vi "3D Surface Graph.vi"() -> ()   [LabVIEW 2014]
doc: "本VI说明了三维曲面的使用方式。"
uses:
  <vilib>/Math Plots/3D Math Plots/3D Surface/3D Surface XCtrl/3D Surface.xctl
  <vilib>/Math Plots/3D Math Plots/3D Mesh/3D Mesh XCtrl/3D Mesh.xctl
  <vilib>/Math Plots/3D Math Plots/3D Contour/3D Contour XCtrl/3D Contour.xctl
  <vilib>/Math Plots/3D Math Plots/3D Contour/3D Contour Datatype/Public/Plot Helper (Vector).vi
  <vilib>/Math Plots/3D Math Plots/3D Mesh/3D Mesh Datatype/Public/Plot Helper (Vector).vi
  <vilib>/Math Plots/3D Math Plots/3D Surface/3D Surface Datatype/Public/Plot Helper (Vector).vi
  <vilib>/imath/engines/lvmath2/RunTimeEngine/Managers/WorkSpace/UID Generator.vi
  <vilib>/imath/engines/lvmath2/RunTimeEngine/BuiltInFunctions/max/1 input/NIMS_max(RV).vi
  <instcachedir>/0/NIMS_max(RV)_237633DB1D604D5BA7001287DF3C7957.lvgen/NIMS_max(RV)_237633DB1D604D5BA7001287DF3C7957_002.vi
  <vilib>/imath/engines/lvmath2/RunTimeEngine/BuiltInFunctions/min/1 input/NIMS_min(RV).vi
  <instcachedir>/0/NIMS_min(RV)_EE2DD3E2888846108C5160A664B67832.lvgen/NIMS_min(RV)_EE2DD3E2888846108C5160A664B67832_002.vi
  <vilib>/imath/engines/lvmath2/RunTimeEngine/BuiltInFunctions/linramp/NIMS_linramp.vi
  <vilib>/imath/engines/lvmath2/RunTimeEngine/BuiltInFunctions/meshgrid2d/NIMS_meshgrid2d(V,V).vi
  <instcachedir>/0/NIMS_meshgrid2d(V,V)_3733343E1C554A708015CFB0432C6A59.lvgen/NIMS_meshgrid2d(V,V)_3733343E1C554A708015CFB0432C6A59_000.vi
  <vilib>/imath/engines/lvmath2/RunTimeEngine/BuiltInFunctions/intrp2d_uneven/NIMS_[1o]_intrp2d_uneven.vi
  <vilib>/imath/engines/lvmath2/RunTimeEngine/RunTimeType/NIMS_RunTimeType_From StrictType (excl LVString).vi
  <instcachedir>/0/NIMS_RunTimeType_From StrictType (excl LVString)_15A5391EEA9C4AACB9955AC755B83D29.lvgen/NIMS_RunTimeType_From StrictType (excl LVString)_15A5391EEA9C4AACB9955AC755B83D29_000.vi
  <vilib>/imath/engines/lvmath2/RunTimeEngine/ErrorHandling/NIMS_Error From Error Code.vi
  <vilib>/imath/engines/lvmath2/RunTimeEngine/LocalVariableDefStatement/MC_LocalVariableDefStatement_Display.vi
  <vilib>/imath/engines/lvmath2/RunTimeEngine/BuiltInFunctions/mesh/NIMS_mesh(RM, RM).vi
  <vilib>/imathl/engines/lvmath/Functions/Error Handling/Create Error.vi
  <vilib>/imath/engines/lvmath2/RunTimeEngine/BuiltInFunctions/grid/NIMS_grid(Enums).vi
  <vilib>/imath/engines/lvmath2/RunTimeEngine/Managers/SymbolTable/Clear UID.vi
  <vilib>/imath/engines/lvmath2/RunTimeEngine/ErrorHandling/NIMS_Finalize Error.vi
  <vilib>/Math Plots/3D Math Plots/3D Surface/3D Surface Datatype/3D Surface Datatype.lvclass
  <vilib>/imath/engines/lvmath2/RunTimeEngine/RangeToken/NIMS_Range_R2 - Integer.vi
  <vilib>/imath/engines/lvmath2/RunTimeEngine/IndexRead/NIMS V(S).vi
  <vilib>/imath/engines/lvmath2/RunTimeEngine/VariableToken/NIMS_VariableToken_CondDefinedDefinedByReplace.vi
  <vilib>/imath/engines/lvmath2/RunTimeEngine/IndexReplace/NIMS M(S,S)=S.vi
  <vilib>/imath/engines/lvmath2/RunTimeEngine/ErrorHandling/NIMS_Create Error From Enums.vi
  <vilib>/imath/engines/lvmath2/RunTimeEngine/CommandStatement/MC_CommandStatement_break.vi
  <vilib>/imath/engines/lvmath2/RunTimeEngine/VariableToken/NIMS_VariableToken_CondDefined.vi
  <vilib>/imath/engines/lvmath2/RunTimeEngine/Managers/SymbolTable/NIMS_WorkSpace.lvlib
  <vilib>/Math Plots/3D Math Plots/3D Mesh/3D Mesh Datatype/3D Mesh Datatype.lvclass
  <vilib>/Math Plots/3D Math Plots/3D Contour/3D Contour Datatype/3D Contour Datatype.lvclass
panel:
  out "3D Contour":refnum<class "3D Plot Datatype.lvclass">[](xcontrol) caption="三维等高线"
  out "3D Mesh":refnum<class "3D Plot Datatype.lvclass">[](xcontrol) caption="三维网格"
  out "ZZ":sgl[][](array[numeric])
  out "Z":sgl[](array[numeric])
  out "Y":i32[](array[numeric])
  out "X":i32[](array[numeric])
  out "三维曲面":refnum<class "3D Plot Datatype.lvclass">[](xcontrol)
  # "e"
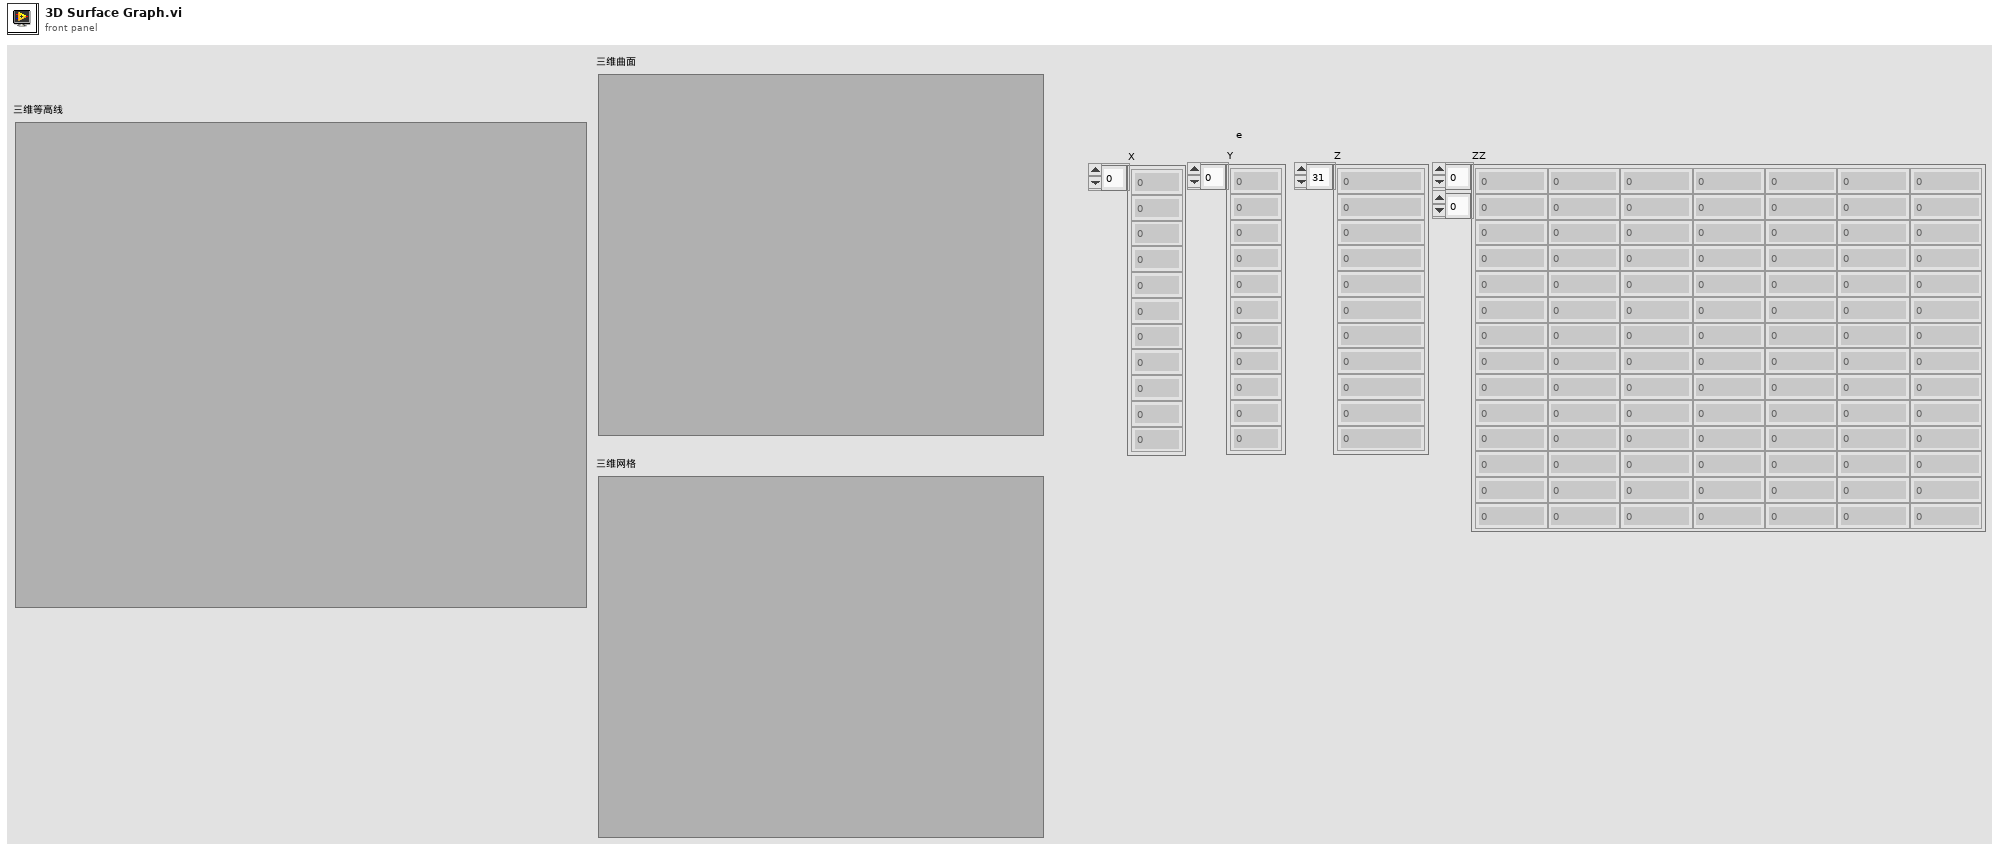
[diagram p1: front panel]
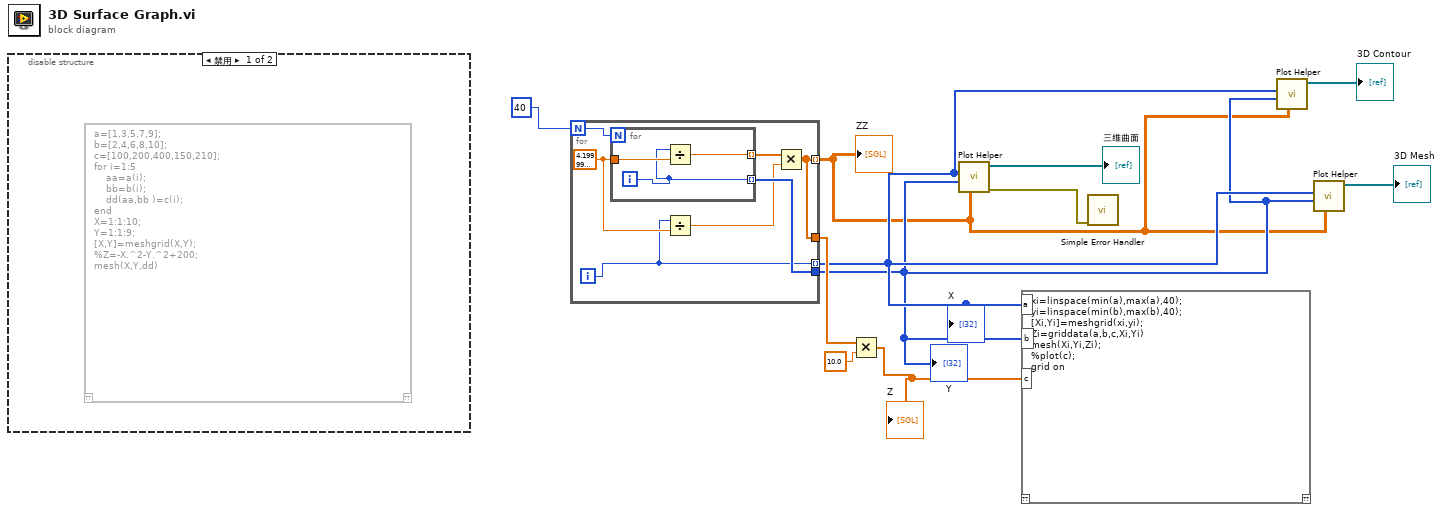
[diagram p0: block diagram]
diagram:
  n1 = disable-structure shown="禁用" {
    frame Disabled {
      n2 = mathscript code="a=[1,3,5,7,9];\nb=[2,4,6,8,10];\nc=[100,200,400,150,210];\nfor i=1:5\n    aa=a(i);\n    bb=b(i);\n    dd(aa,bb )=c(i);\nend\nX=1:1:10;\nY=1:1:9;\n[X,Y]=meshgrid(X,Y);\n%Z=-X.^2-Y.^2+200;\nmesh(X,Y,dd)"() -> ()  [unwired: 1 in, 1 out]
    }
    frame Enabled {
    }
  }
  n3 = for {
    N: 40 ("X input length") -> [w213]
    tunnel: [w210] -> w1 mode=indexing
    tunnel: [w208] -> w3 mode=indexing
    tunnel: [w211] -> w2
    tunnel: [w210] -> w8
    i -> [w208]
    w212 = sgl 4.2 ("y")
    n4 = for {
      N: w213 -> [_]
      tunnel: [w216] -> w214 mode=indexing
      tunnel: w212 -> [w217]
      tunnel: [w215] -> w211 mode=indexing
      i -> [w215]
      n5 = Divide(x=w215, y=w217) -> (x/y=w216:sgl)
    }
    n6 = Divide(x=w208, y=w212) -> (x/y=w209:sgl)
    n7 = Multiply(x=w214, y=w209) -> (x*y=w210:sgl[])
  }
  "X" <- w3
  "Y" <- w2
  "ZZ" <- w1
  n8 = Multiply(x=w8, y=10.0) -> (x*y=w6:dbl[])
  "Z" <- w6
  n9 = call-poly <vilib>:"Plot Helper.vi"("z matrix"=w1, "y vector"=w2, "x vector"=w3) -> ("error out"=w10:errorcluster, "3D Plot lvclass Array out"=→"三维曲面":refnum<class "3D Plot Datatype.lvclass">[])  [unwired: 4 in, 3 out]
  n10 = mathscript code="xi=linspace(min(a),max(a),40);\nyi=linspace(min(b),max(b),40);\n[Xi,Yi]=meshgrid(xi,yi);\nZi=griddata(a,b,c,Xi,Yi)\nmesh(Xi,Yi,Zi);\n%plot(c);\ngrid on"("a"=w3, "b"=w2, "c"=w6) -> ()  [unwired: 1 in, 1 out]
  n11 = call <vilib>:"Simple Error Handler.vi"("error in (no error)"=w10) -> ()  [unwired: 4 in, 5 out]
  n12 = call-poly <vilib>:"Plot Helper.vi"("z matrix"=w1, "y vector"=w2, "x vector"=w3) -> ("3D Plot lvclass Array out"=→"3D Contour":refnum<class "3D Plot Datatype.lvclass">[])  [unwired: 3 in, 5 out]
  n13 = call-poly <vilib>:"Plot Helper.vi"("z matrix"=w1, "y vector"=w2, "x vector"=w3) -> ("3D Plot lvclass Array out"=→"3D Mesh":refnum<class "3D Plot Datatype.lvclass">[])  [unwired: 3 in, 5 out]
